vi "RT_Config_sbRIO.vi"() -> (0 "error out":errorcluster, 3 "FPGA VI Reference Out":refnum<k20>)   [LabVIEW 2011]
uses:
  <vilib>/rvi/interface/nirviMethod/nirviMethod.xnode
  <vilib>/rvi/interface/nirviOpenFPGA/nirviOpenFPGA.xnode
  <vilib>/FPGAPlugInAG/Dynamic/niLvFpga_StartFifo_Dynamic.vi
  <vilib>/rvi/errors/niLvFpgaMergeErrorWithErrorCode.vi
  <vilib>/FPGAPlugInAG/Dynamic/niLvFpga_AcknowledgeIrq_Dynamic.vi
  <vilib>/rvi/interface/nirviMethod/StockFPGA_InlinedMethodWaitForSingleIRQ.vi
  <vilib>/FPGAPlugInAG/Dynamic/niLvFpga_WaitOnIrq_Dynamic.vi
  FPGA Bitfiles/RSProject1_FPGATarget_FPGAsbFOGv3_VB7HW11FQ7c.lvbitx
  <vilib>/LabVIEW Targets/FPGA/cRIO/shared/nicrio_ModuleControls/nicrio_cRIO-9871_BaudRateEnum.ctl
  <vilib>/rvi/interface/nirviReadWriteControl/nirviReadWriteControl.xnode
  <vilib>/FPGAPlugInAG/Dynamic/niLvFpga_Reset_Dynamic.vi
  <vilib>/rvi/interface/Simulation/niFpgaSimulationCallBeginRW.vi
  <vilib>/rvi/errors/niLvFpgaAdjustHostInterfaceError.vi
  <vilib>/FPGAPlugInAG/Dynamic/niLvFpga_Run_Dynamic.vi
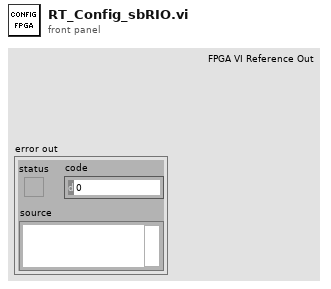
[diagram p1: front panel]
types:
  T1 = typedef "nicrio_cRIO-9871_BaudRateEnum.ctl" = enum16{"75 bps", "110 bps", "134 bps", "150 bps", "300 bps", "600 bps", "1200 bps", "1800 bps", "2400 bps", "4800 bps", "7200 bps", "9600 bps", "14.4 kbps", "19.2 kbps", "28.8 kbps", "38.4 kbps", "57.6 kbps", "115.2 kbps", "230.4 kbps", "460.8 kbps", "921.6 kbps"}
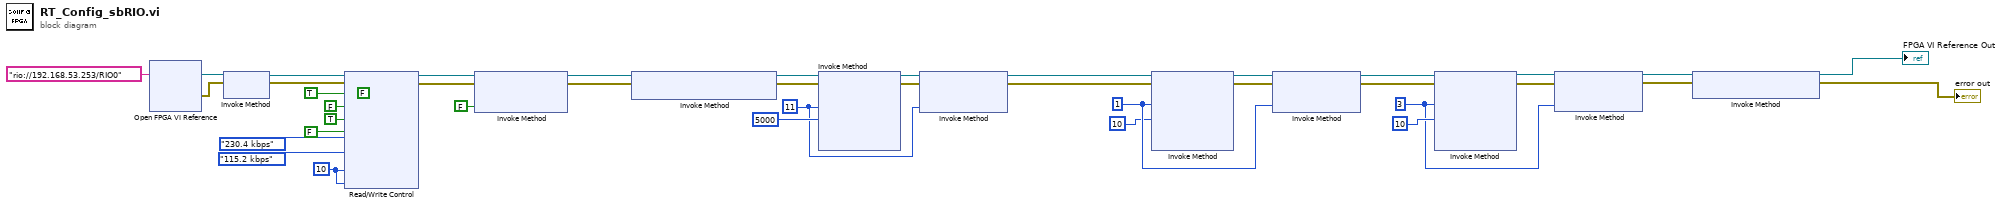
[diagram p0: block diagram]
diagram:
  w7 = 11 ("IRQ Number(s)")
  w19 = 1 ("IRQ Number(s)")
  w22 = 3 ("IRQ Number(s)")
  w13 = 10 ("Timeout_FR 1")
  (unwired) FALSE ("Port1?")
  n1 = xnode "Open FPGA VI Reference"("resource name"=tag "rio://192.168.53.253/RIO0") -> ("FPGA VI Reference Out"=w28:refnum<k20>, "error out"=w29:errorcluster)  [unwired: 1 in]
  n2 = xnode "Invoke Method"("FPGA VI Reference In"=w28, "error in"=w29) -> ("FPGA VI Reference Out"=w34:refnum<k20>, "error out"=w35:errorcluster)
  n3 = xnode "Read/Write Control"("FPGA VI Reference In"=w34, "error in"=w35, "Port1?"=TRUE, "Port4?"=FALSE, "Port3?"=TRUE, "Port2?"=FALSE, "Baud Rate_P1"=nicrio_cRIO-9871_BaudRateEnum."230.4 kbps", "Baud Rate_P3"=nicrio_cRIO-9871_BaudRateEnum."115.2 kbps", "Timeout_FW 3"=w13, "Timeout_PW 3"=w13) -> ("FPGA VI Reference Out"=w32:refnum<k20>, "error out"=w33:errorcluster)
  n4 = xnode "Invoke Method"("FPGA VI Reference In"=w32, "error in"=w33, "Wait Until Done (F)"=FALSE) -> ("FPGA VI Reference Out"=w6:refnum<k20>, "error out"=w5:errorcluster)
  n5 = xnode "Invoke Method"("FPGA VI Reference In"=w6, "error in"=w5) -> ("FPGA VI Reference Out"=w11:refnum<k20>, "error out"=w12:errorcluster)
  n6 = xnode "Invoke Method"("FPGA VI Reference In"=w11, "error in"=w12, "IRQ Number(s)"=w7, "Timeout (ms)"=5000) -> ("FPGA VI Reference Out"=w9:refnum<k20>, "error out"=w10:errorcluster)  [unwired: 2 out]
  n7 = xnode "Invoke Method"("FPGA VI Reference In"=w9, "error in"=w10, "IRQ Number(s)"=w7) -> ("FPGA VI Reference Out"=w4:refnum<k20>, "error out"=w3:errorcluster)
  n8 = xnode "Invoke Method"("FPGA VI Reference In"=w4, "error in"=w3, "IRQ Number(s)"=w19, "Timeout (ms)"=10) -> ("FPGA VI Reference Out"=w17:refnum<k20>, "error out"=w16:errorcluster)  [unwired: 2 out]
  n9 = xnode "Invoke Method"("FPGA VI Reference In"=w17, "error in"=w16, "IRQ Number(s)"=w19) -> ("FPGA VI Reference Out"=w15:refnum<k20>, "error out"=w14:errorcluster)
  n10 = xnode "Invoke Method"("FPGA VI Reference In"=w15, "error in"=w14, "IRQ Number(s)"=w22, "Timeout (ms)"=10) -> ("FPGA VI Reference Out"=w21:refnum<k20>, "error out"=w20:errorcluster)  [unwired: 2 out]
  n11 = xnode "Invoke Method"("FPGA VI Reference In"=w21, "error in"=w20, "IRQ Number(s)"=w22) -> ("FPGA VI Reference Out"=w24:refnum<k20>, "error out"=w25:errorcluster)
  n12 = xnode "Invoke Method"("FPGA VI Reference In"=w24, "error in"=w25) -> ("FPGA VI Reference Out"=→"FPGA VI Reference Out":refnum<k20>, "error out"=→"error out":errorcluster)
